vi "aggregator - vi - real - atomic.vi"(5 "aggregator action":T1, 6 "init?":bool, 7 "requested size":i32=20, 8 "number":dbl, 11 "state IN":T2={"requested size"=20, "Array"=[], "actual number of elements"=0}) -> (0 "slope":dbl, 1 "interp average":dbl, 2 "mean":dbl, 3 "state OUT":T2={"requested size"=20, "Array"=[], "actual number of elements"=0})   [LabVIEW 2015]
uses:
  interpolation state - real.ctl
  agregator -- action.ctl
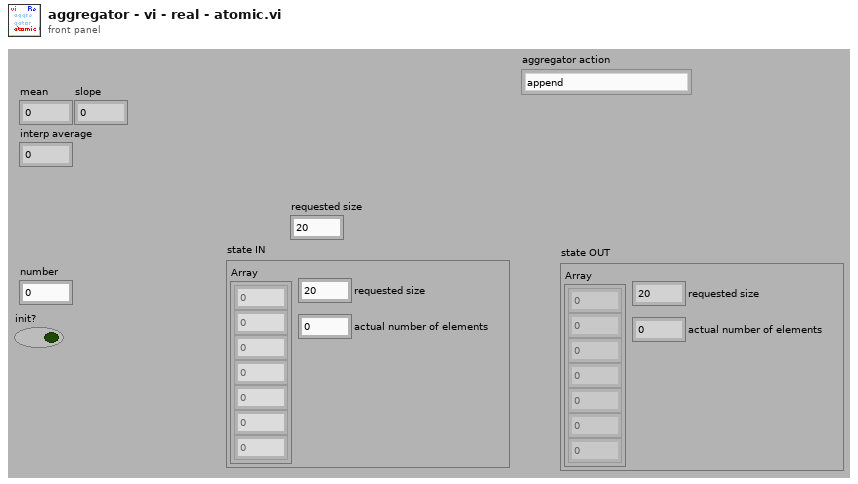
[diagram p1: front panel]
types:
  T1 = typedef "agregator -- action.ctl" = enum16{"append", "interpolate", "empty!", "force"}
  T2 = typedef "interpolation state - real.ctl" = cluster{"requested size":i32, "Array":dbl[], "actual number of elements":i32}
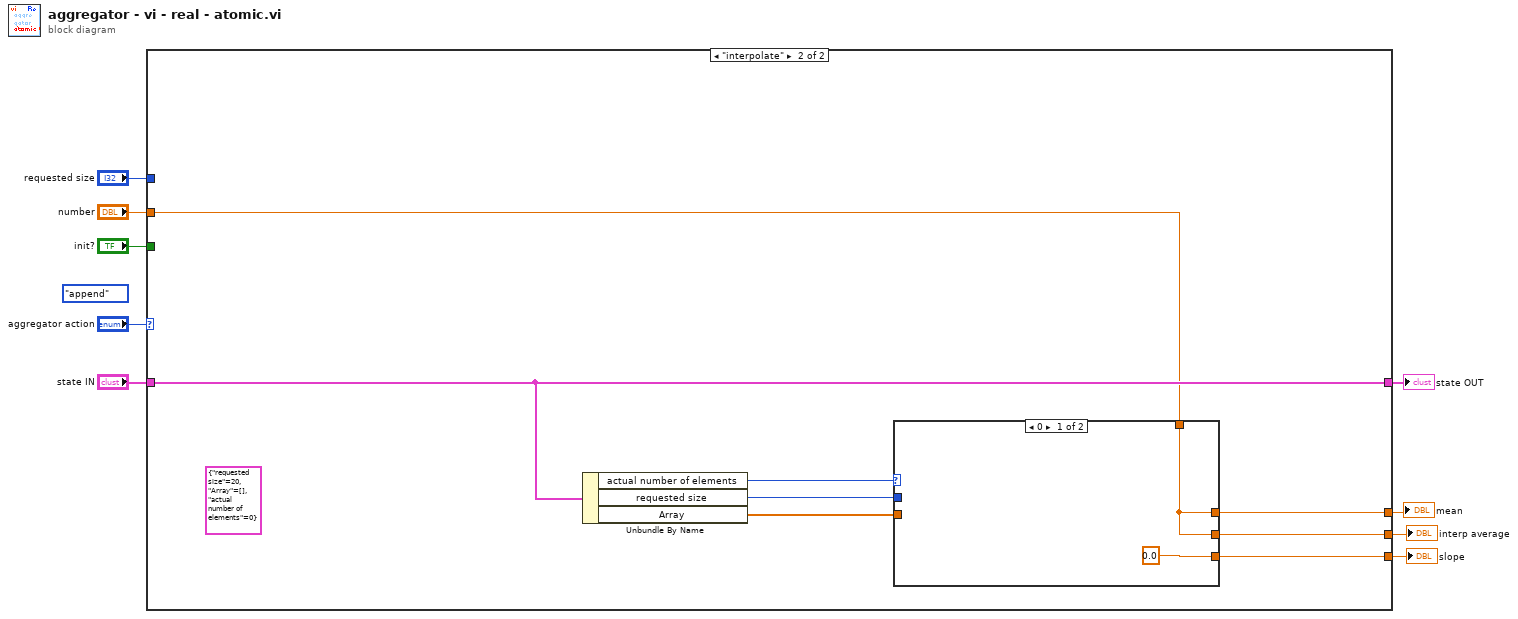
[diagram p0: block diagram]
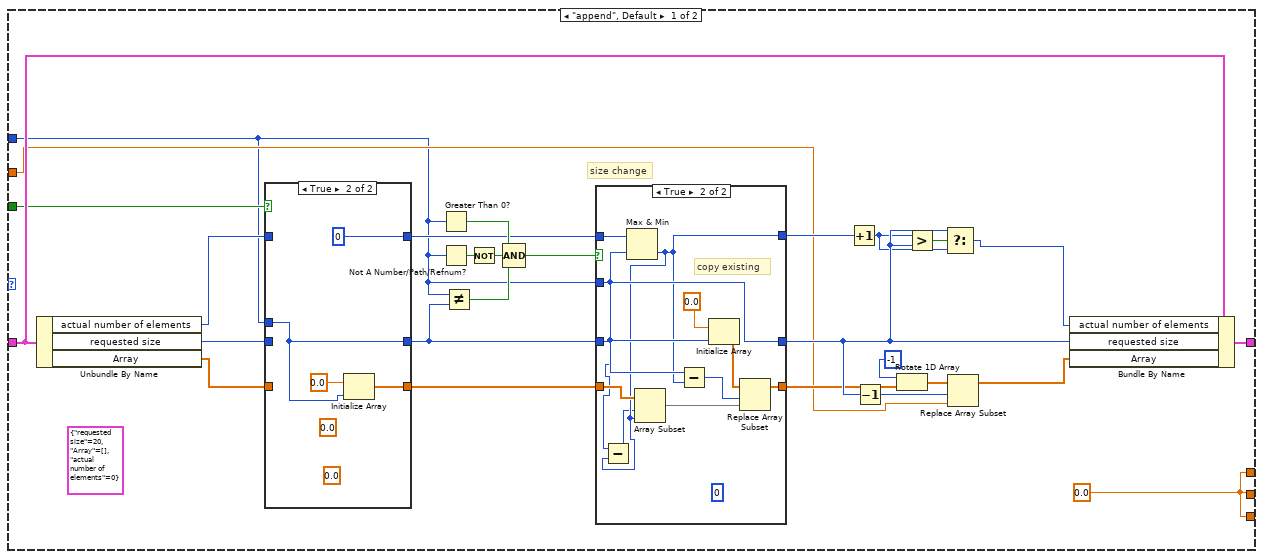
[diagram p2: hidden frame]
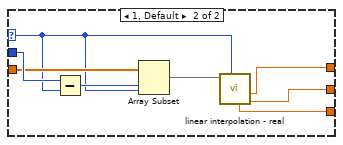
[diagram p5: hidden frame]
diagram:
  (unwired) agregator_--_action."append" ("aggregator action")
  n1 = case shown="\"interpolate\"" "aggregator action" {
    tunnel: [w13 w65] -> w9
    tunnel: [w13 w64] -> w8
    tunnel: [w13 w63] -> w7
    tunnel: [w33 w59] -> w6
    tunnel: "state IN" -> [w32 w59]
    tunnel: "init?" -> [w12 _]
    tunnel: "number" -> [w11 w58]
    tunnel: "requested size" -> [w10 _]
    frame "append", Default {
      w13 = 0.0 ("mean")
      (unwired) T2 {"requested size"=20, "Array"=[], "actual number of elements"=0} ("Cluster")
      # "size change"
      n2 = Unbundle By Name(w32) -> ("actual number of elements"=w35:i32, "requested size"=w36:i32, "Array"=w34:dbl[])
      n3 = case shown="True" w12 {
        tunnel: w35 -> [w53 _]
        tunnel: [w53 0] -> w18
        tunnel: w34 -> [w51 _]
        tunnel: w10 -> [_ w54]
        tunnel: w36 -> [w52 _]
        tunnel: [w51 w55] -> w21
        tunnel: [w52 w54] -> w19
        frame False {
        }
        frame True {
          (unwired) 0.0
          (unwired) 0.0
          n4 = Initialize Array(0.0, w54) -> (w55:dbl[])
        }
      }
      n5 = Greater Than 0?(x=w10) -> (x > 0?=w25:bool)
      n6 = Not A Number/Path/Refnum?(number/path/refnum=w10) -> (NaN/Path/Refnum?=w26:bool)
      n7 = Not Equal?(x=w10, y=w19) -> (x != y?=w23:bool)
      n8 = Not(x=w26) -> (.not. x?=w24:bool)
      n9 = Compound Arithmetic op=AND(w25, w24, w23) -> (w22:bool)
      n10 = case shown="True" w22 {
        tunnel: [w39 w41] -> w17
        tunnel: w18 -> [w39 w49]
        tunnel: [w38 w45] -> w30
        tunnel: w19 -> [w38 w42]
        tunnel: [w37 w48] -> w20
        tunnel: w21 -> [w37 w44]
        tunnel: w10 -> [_ w45]
        frame False {
        }
        frame True {
          (unwired) 0 ("disabled index (col)")
          # "copy existing"
          n11 = Max & Min(x=w49, y=w45) -> (min(x,y)=w41:i32)  [unwired: 1 out]
          n12 = Subtract(x=w42, y=w41) -> (x-y=w40:i32)
          n13 = Array Subset(array=w44, index=w40, length=w41) -> (w43:dbl[])
          n14 = Subtract(x=w45, y=w41) -> (x-y=w46:i32)
          n15 = Initialize Array(0.0, w45) -> (w47:dbl[])
          n16 = Replace Array Subset(array=w47, new element=w43, index=w46) -> (w48:dbl[])
        }
      }
      n17 = Increment(x=w17) -> (x+1=w27:i32)
      n18 = Decrement(x=w30) -> (x-1=w15:i32)
      n19 = Rotate 1D Array(1:w20, 2:-1 ("n")) -> (0:w14:dbl[])
      n20 = Greater?(x=w27, y=w30) -> (0:w28:bool)
      n21 = Select(t=w30, s=w28, f=w27) -> (s? t:f=w31:i32)
      n22 = Replace Array Subset(array=w14, new element=w11, index=w15) -> (w29:dbl[])
      n23 = Bundle By Name(cluster=w32, "actual number of elements"=w31, "requested size"=w30, "Array"=w29) -> (w33:T2)
    }
    frame "interpolate" {
      (unwired) T2 {"requested size"=20, "Array"=[], "actual number of elements"=0} ("Cluster")
      n24 = Unbundle By Name(w59) -> ("actual number of elements"=w60:i32, "requested size"=w62:i32, "Array"=w61:dbl[])
      n25 = case shown="0" w60 {
        selector: w60 -> [_ w68]
        tunnel: [w66 w75] -> w65
        tunnel: [w66 w74] -> w64
        tunnel: [0.0 w73] -> w63
        tunnel: w62 -> [_ w72]
        tunnel: w61 -> [_ w71]
        tunnel: w58 -> [w66 _]
        frame 0 {
        }
        frame 1, Default {
          n26 = Subtract(x=w72, y=w68) -> (x-y=w70:i32)
          n27 = Array Subset(array=w71, index=w70, length=w68) -> (w69:dbl[])
          n28 = call "linear interpolation - real.vi"("n"=w68, "Array"=w69) -> ("interpolated average"=w74:dbl, "mean"=w75:dbl, "slope"=w73:dbl)  [unwired: 4 in, 3 out]
        }
      }
    }
  }
  "mean" <- w9
  "interp average" <- w8
  "slope" <- w7
  "state OUT" <- w6
